vi "z shm client new.vi"(8 "error in (no error)":errorcluster, 9 "callbacks":cluster{}, 10 "context":cluster{"ptr":u64}, 11 "this_":cluster{}) -> (0 "error out":errorcluster, 3 "this_ out":cluster{})   [LabVIEW 2021, in "zenohc.lvlib"]
doc: "void z_shm_client_new(struct z_owned_shm_client_t *this_,\n struct zc_threadsafe_context_t context,\n struct zc_shm_client_callbacks_t callbacks);"
uses:
  zenohc.lvlib
  zenohc.dll
  <resource>/importtools/sharedlib/VI/Block Diagram/Call Library Node/Call Library Node.lvlib
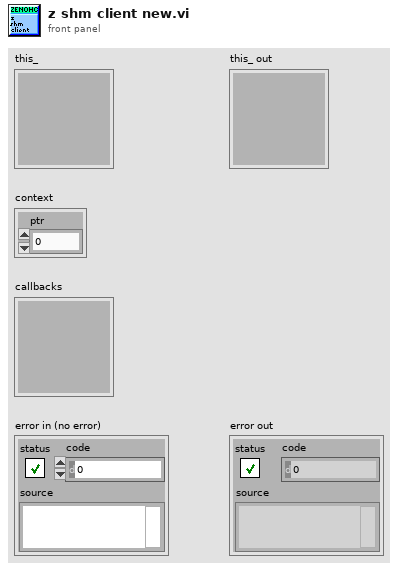
[diagram p1: front panel]
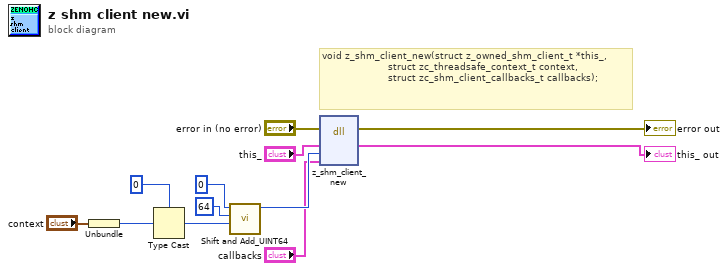
[diagram p0: block diagram]
diagram:
  # "void z_shm_client_new(struct z_owned_shm_client_t *this_,\n                      struct zc_threadsafe_context_t context,\n                      struct zc_shm_client_callbacks_t callbacks);"
  n1 = Unbundle("context") -> ("ptr"=w9:u64)
  n2 = Type Cast(type=u64 0, x=w9) -> (*(type *) &x=w7:u64)
  n3 = call <resource>:"Shift and Add_UINT64.vi"("Add Num"=w7, "shift bits"=64, "Shift Num"=u64 0) -> ("Result"=w4:u64)  [unwired: 8 in]
  n4 = dll-call lib="D:/dev/zenoh_labview/zenohc/zenohc.*" fn="z_shm_client_new"(error in="error in (no error)", "this_"="this_", "context"=w4, "callbacks"="callbacks") -> (error out=→"error out":errorcluster, "this_"=→"this_ out":cluster{})  [unwired: 5 in, 1 out]
